vi "Main.vi"(8 "error in":errorcluster, 11 "Maestro Control in":refnum<class "Maestro Control.lvclass">) -> (0 "error out":errorcluster, 3 "Maestro Control out":refnum<class "Maestro Control.lvclass">)   [LabVIEW 2021, in "Maestro Control.lvclass"]
doc: "The Queued Message Handler of a Worker."
uses:
  Maestro Control.lvclass
  C:/Program Files (x86)/National Instruments/LabVIEW 2021/vi.lib/addons/_Workers/Library/Classes/Worker/Worker.lvclass
  Maestro Control.lvclass/Maestro Control.ctl
  <vilib>/addons/_Workers/Library/Classes/Worker/Worker.lvclass/Worker.ctl
  UI State.ctl
  85a54a2c-5f55-4a01-b73e-4297187ed6bb.vi
  85a54a2c-5f55-4a01-b73e-4297187ed6bb.vi/659df739-fa42-474c-bf03-f9ba45f35773.vi
  Maestro Acq/Maestro Acq.lvclass
  Maestro Data Logg/Maestro Data Logg.lvclass
  <userlib>/LV-TOML/lib/Parse TOML String.vi
  <userlib>/LV-TOML/lib/TOML to LabVIEW.vi
  <vilib>/addons/_Workers/Library/Classes/Message/Enqueue Message to Self v2.vi
  <userlib>/LV-TOML/lib/Write TOML File (TOML).vi
  <vilib>/addons/_Workers/Library/Classes/Message/Enqueue Message to Queue.vi
  Initialization Data.ctl
  <vilib>/addons/_Workers/Library/Classes/Worker/Worker.lvclass
  <vilib>/addons/_Workers/Debugger/Debug Client/Debug Client.lvlib
  <vilib>/addons/_Workers/Library/Classes/Message/Message.lvclass
  <userlib>/LV-TOML/lib/LV-TOML.lvlib
  C:/Program Files (x86)/National Instruments/LabVIEW 2021/vi.lib/addons/_Workers/Library/Classes/Workers Object/Workers Object.lvclass
  C:/Users/flepetit/Desktop/Gentec-maestro-Labview/Workers/Maestro Control/Maestro Control.lvclass
  C:/Users/flepetit/Desktop/Gentec-maestro-Labview/Workers/Maestro Acq/Maestro Acq.lvclass
  C:/Users/flepetit/Desktop/Gentec-maestro-Labview/Workers/Maestro Data Logg/Maestro Data Logg.lvclass
panel:
  in  "Activer les Stats":bool
  out "Maestro Online":bool
  in  "disconnect":bool
  in  "connect":bool
  in  "Port":i16
  in  "Adress(ip)":string
  out "Datas":waveform(dbl)[](graph)
  in  "délai d'acq.(ms)":i32
  in  "Log File Path":path
  out "Puiss.":dbl format="%#_6e"
  in  "Stop":bool
  in  "Start":bool
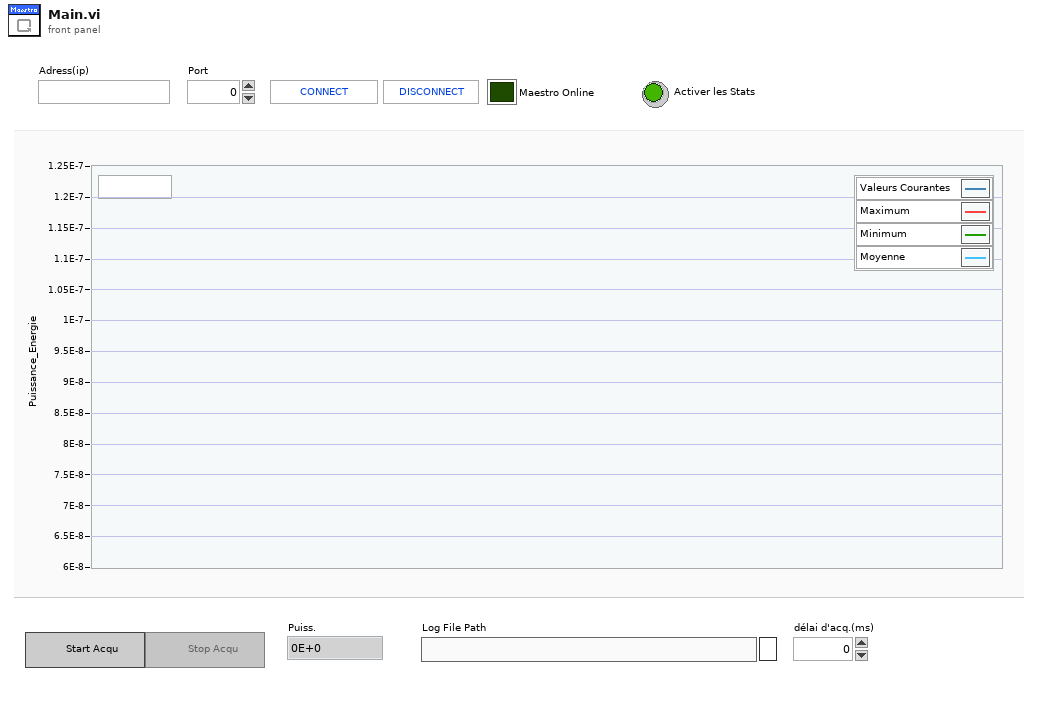
[diagram p1: front panel]
types:
  T1 = cluster{"Tps(s)":dbl[], "Puiss.":dbl, "Waveform":waveform(dbl)[]}
  T2 = enum16{"open", "replace", "create", "open or create", "replace or create", "replace or create with confirmation"}
  T3 = typedef "Maestro Control.lvclass/Initialization Data.ctl" = cluster{"String":string}
  T4 = typedef "Maestro Control.lvclass/UI State.ctl" = enum16{"Idle", "Acquiring and Logging", "Waiting for Exit", "Waiting for Exit (Acq Stopped)", "Waiting for Exit (Log Stopped)", "Waiting for Stop", "Waiting for Stop (Acq Stopped)", "Waiting for Stop (Log Stopped)"}
  T5 = typedef "Maestro Acq.lvclass/Hardware Maestro Config.ctl" = cluster{"Adress(ip)":string, "Port":i16, "Log File Base Path":path, "délai d'acq.(ms)":i32, "Activer les Stats":bool}
  T6 = typedef "Workers.lvlib/Case Label.ctl" = string
  T7 = typedef "LV-TOML.lvlib/TOML Value.ctl" = cluster{"type":enum16{"Table", "Array", "String", "Integer", "Float", "Boolean", "Offset Date-Time", "Local Date-Time", "Local Date", "Local Time", "Path"}, "value":variant}
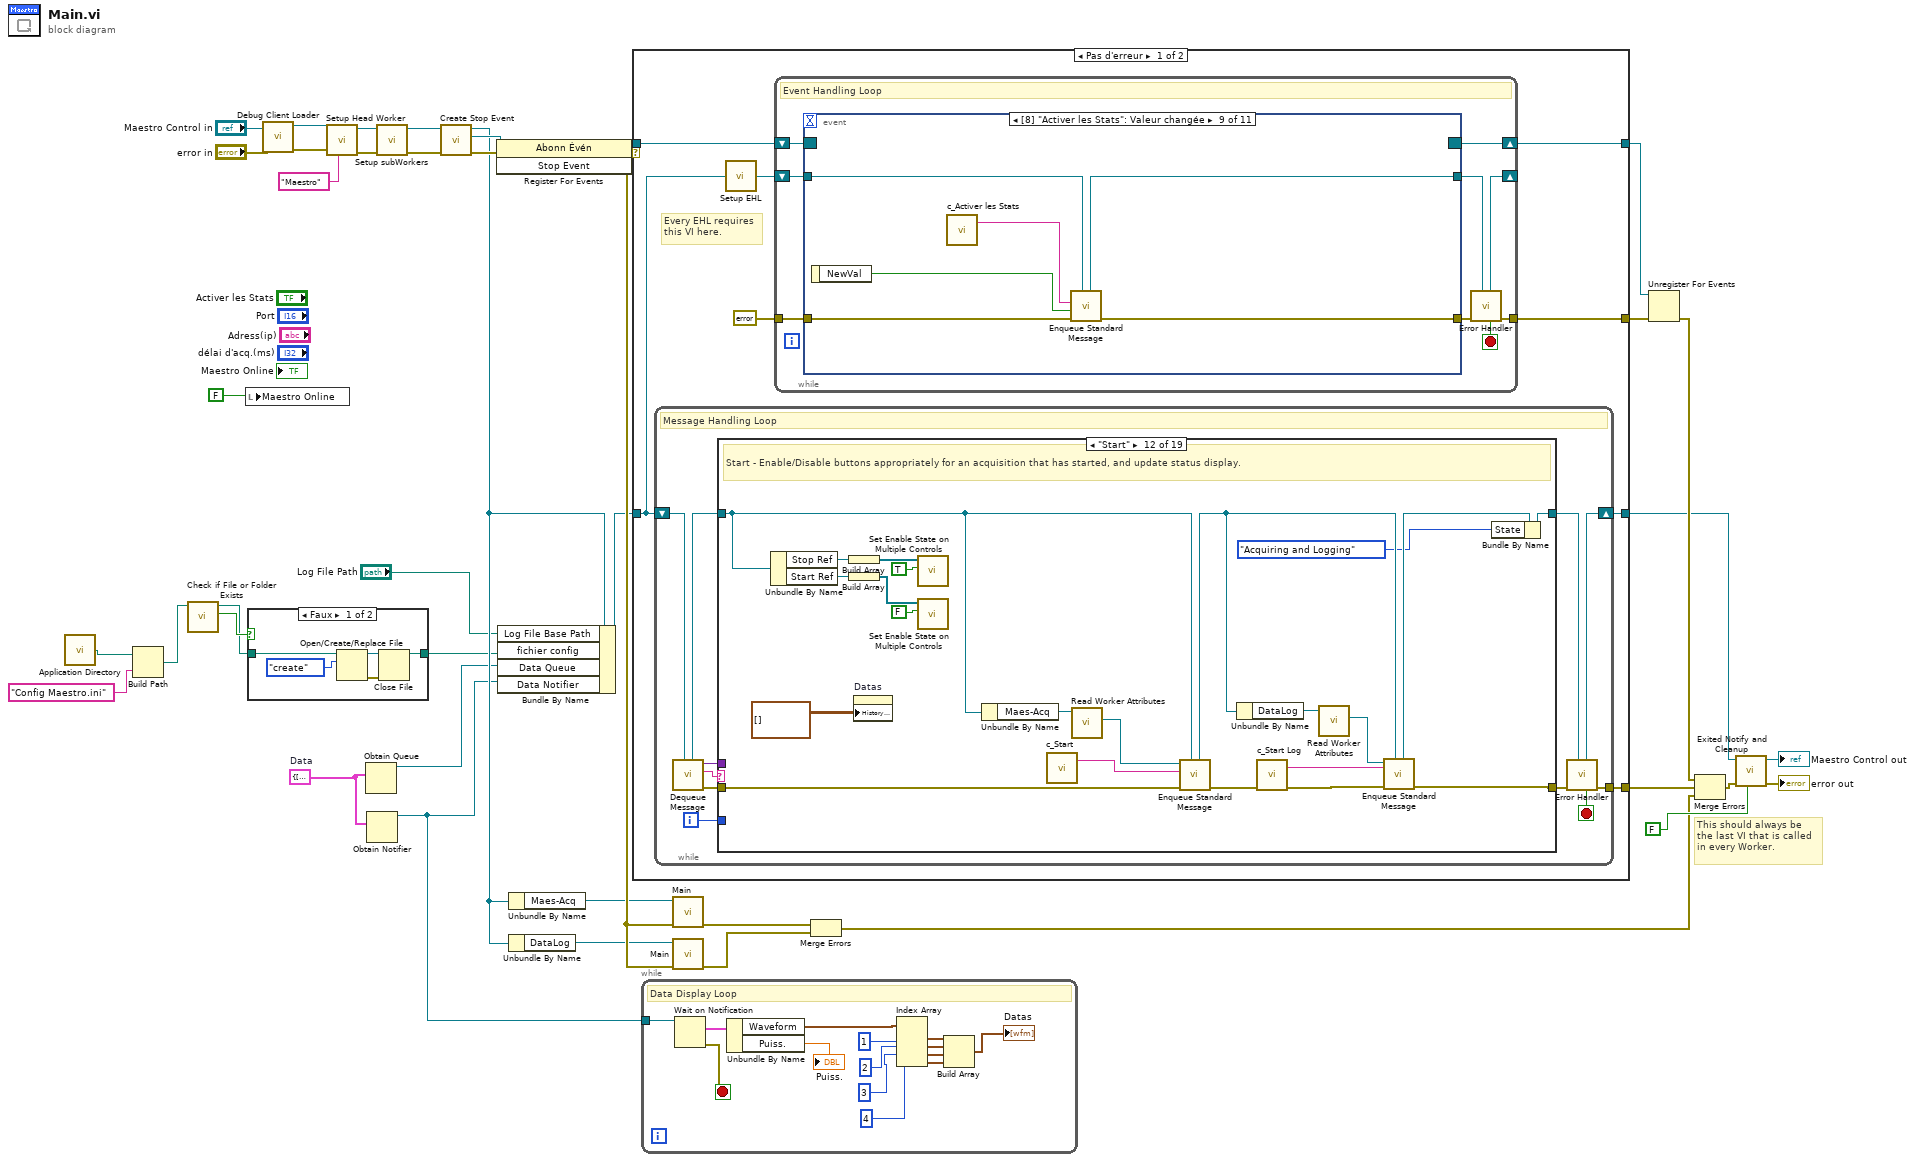
[diagram p0: block diagram]
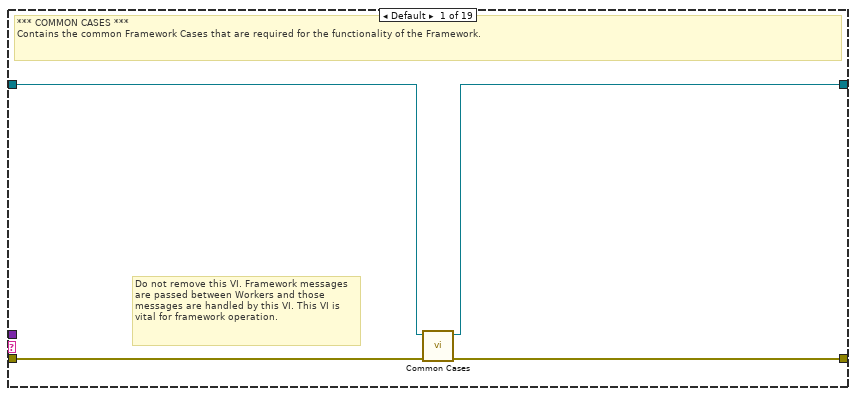
[diagram p3: hidden frame]
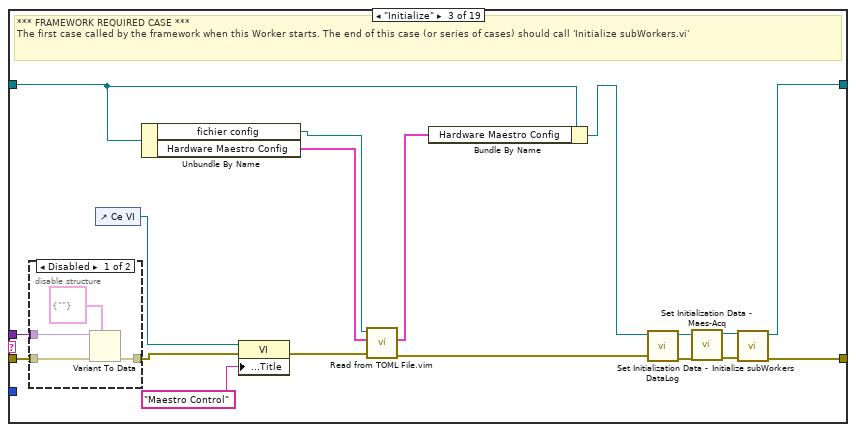
[diagram p5: hidden frame]
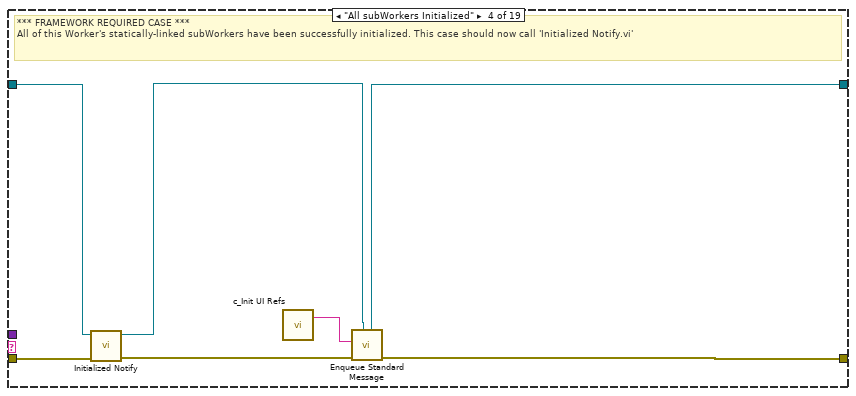
[diagram p7: hidden frame]
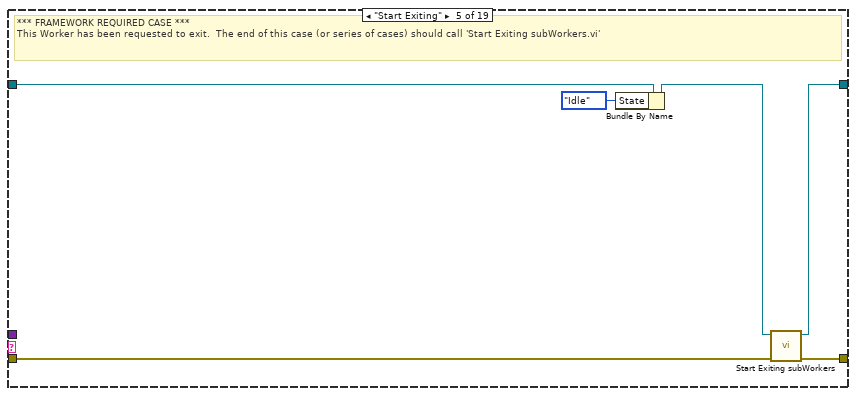
[diagram p8: hidden frame]
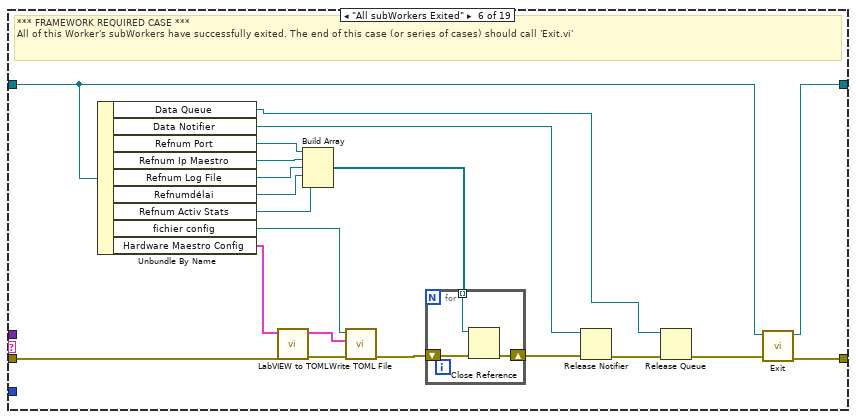
[diagram p9: hidden frame]
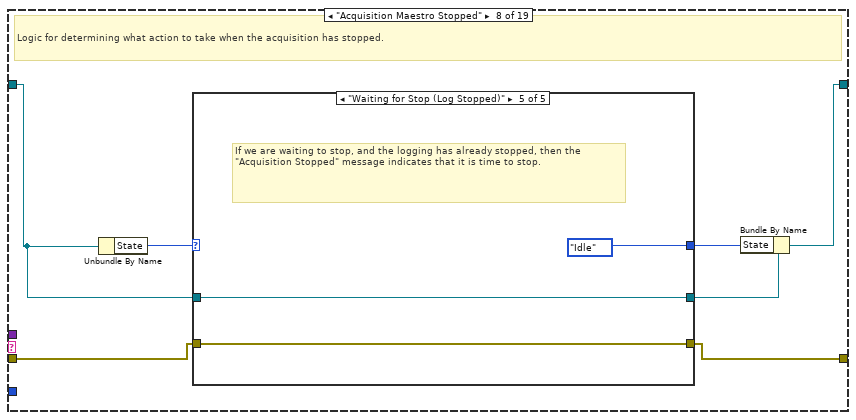
[diagram p11: hidden frame]
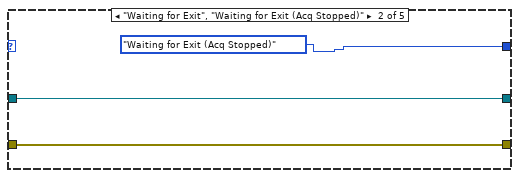
[diagram p13: hidden frame]
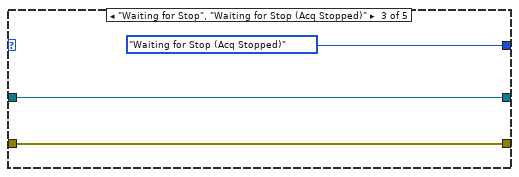
[diagram p14: hidden frame]
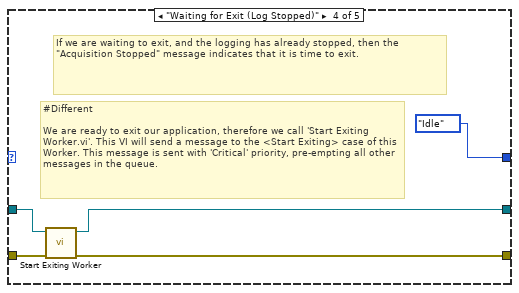
[diagram p15: hidden frame]
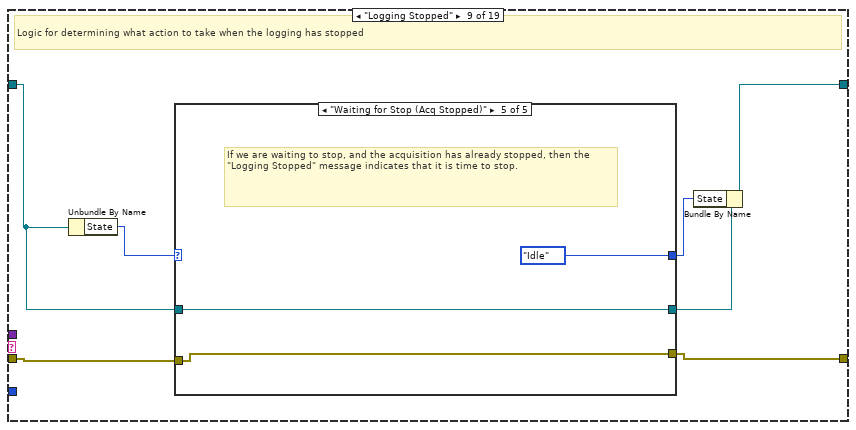
[diagram p16: hidden frame]
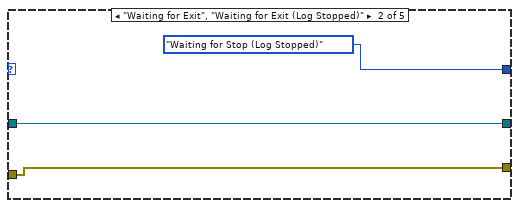
[diagram p18: hidden frame]
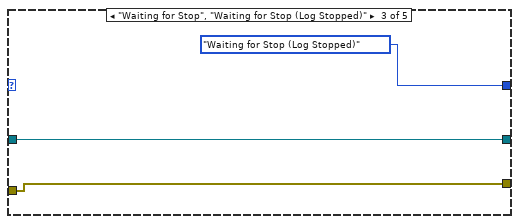
[diagram p19: hidden frame]
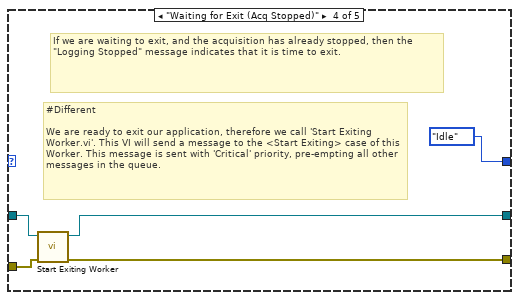
[diagram p20: hidden frame]
diagram:
  w4 = T1 {"Tps(s)"=[], "Puiss."=0.0, "Waveform"=[]}  # Data
  # "This should always be the last VI that is called in every Worker."
  n1 = call <vilib>:"Application Directory.vi"() -> ("Application Directory"=w11:path)
  n2 = Build Path(base path=w11, name or relative path="Config Maestro.ini") -> (appended path=w10:path)
  n3 = call <vilib>:"Check if File or Folder Exists.vi"("path"=w10) -> ("file or folder exists?"=w9:bool, "dup path"=w8:path)  [unwired: 8 in, 1 out]
  n4 = local write "Maestro Online"(FALSE ("connect")) -> ()
  n5 = case "Structure Condition" shown="Faux" w9 {
    tunnel: w8 -> [w45 w46]
    tunnel: [w42 w46] -> w6
    frame False {
      n6 = Open/Create/Replace File(file path (use dialog)=w45, operation (0:open)=T2."create" ("opération (0 : open)")) -> (refnum out=w44:refnum<file>, error out=w43:errorcluster)  [unwired: 4 in, 1 out]
      n7 = Close File(refnum=w44, error in=w43) -> (path=w42:path)  [unwired: 1 out]
    }
    frame True {
    }
  }
  n8 = call <vilib>:"Debug Client Loader.vi"("error in (no error)"="error in", "Worker"="Maestro Control in") -> ("error out"=w19:errorcluster, "Worker out"=w20:refnum<class "Maestro Control.lvclass">)  [unwired: 8 in]
  n9 = call-dynamic "Setup Head Worker.vi"("Worker Alias"="Maestro", "error in"=w19, "Worker"=w20) -> ("error out"=w15:errorcluster, "Worker out"=w18:refnum<class "Maestro Control.lvclass">)  [unwired: 7 in]
  n10 = Obtain Queue(element data type=w4) -> (queue out=w3:refnum<queue>)  [unwired: 4 in, 2 out]
  n11 = Obtain Notifier(notification data type=w4) -> (notifier out=w2:refnum<notifier>)  [unwired: 3 in, 2 out]
  n12 = call "Setup subWorkers.vi"("error in"=w15, "Maestro Control in"=w18) -> ("error out"=w16:errorcluster, "Maestro Control out"=w17:refnum<class "Maestro Control.lvclass">)  [unwired: 8 in]
  n13 = call-dynamic "Create Stop Event.vi"("error in"=w16, "Worker"=w17) -> ("error out"=w35:errorcluster, "Stop Event"=w32:refnum<user-event>, "Worker out"=w29:refnum<class "Maestro Control.lvclass">)  [unwired: 7 in]
  n14 = register-events(error in=w35, w32) -> (reference out=w34:refnum<event-registration>, error out=w28:errorcluster)  [unwired: 1 in]
  n15 = Bundle By Name(cluster=w29, "Log File Base Path"="Log File Path", "fichier config"=w6, "Data Queue"=w3, "Data Notifier"=w2) -> (w7:refnum<class "Maestro Control.lvclass">)
  n16 = Unbundle By Name(w29) -> ("Maes-Acq"=w23:refnum<class "Maestro Acq.lvclass">)
  n17 = Unbundle By Name(w29) -> ("DataLog"=w13:refnum<class "Maestro Data Logg.lvclass">)
  n18 = case shown="Pas d'erreur" w28 {
    tunnel: w7 -> [w49 w379]
    tunnel: [w47 w380] -> w33
    tunnel: w34 -> [w54 w381]
    tunnel: [w51 w382] -> w39
    tunnel: [w53 w381] -> w38
    tunnel: [w48 w378] -> w36
    selector: w28 -> [_ w382]
    frame No Error {
      # "Every EHL requires\nthis VI here."
      n19 = while {
        shift-right: [w63] -> w48
        shift-left: w49 -> [w65]
        tunnel: [w64] -> w47
        i -> [w55]
        stop <- w56 stop-if-true
        # "Message Handling Loop"
        n20 = call-dynamic "Dequeue Message.vi"("Worker"=w65) -> ("error out"=w62:errorcluster, "Case out"=w57:string, "Data out"=w58:variant, "Worker out"=w60:refnum<class "Maestro Control.lvclass">)  [unwired: 6 in, 1 out]
        n21 = case "Worker MHL Case Structure (DO NOT CHANGE LABEL NAME)" shown="\"Start\"" w57 {
          tunnel: w62 -> [w69 w70 w87 w100 w104 w124 w131 w138 w158 w185 w187 w207 w215 w222 w233 w245 w262 w282 w293]
          tunnel: [w68 w70 w89 w98 w107 w127 w131 w137 w157 w183 w187 w197 w210 w218 w230 w241 w249 w270 w292] -> w61
          tunnel: w60 -> [w67 w71 w81 w101 w105 w125 w132 w139 w162 w186 w188 w199 w216 w223 w234 w246 w263 w276 w302]
          tunnel: [w66 w71 w88 w96 w106 w126 w132 w135 w163 w186 w188 w191 w212 w220 w225 w240 w253 w267 w290] -> w59
          tunnel: w58 -> [_ _ w86 _ _ _ _ _ _ w184 _ _ w214 w221 w232 w244 w261 _ _]
          tunnel: w55 -> [_ _ _ _ _ _ _ _ _ _ _ _ _ _ _ _ _ _ _]
          frame Default {
            # "Do not remove this VI. Framework messages are passed between Workers and those messages are handled by this VI. This VI is vital for framework operation."
            # "*** COMMON CASES ***\nContains the common Framework Cases that are required for the functionality of the Framework."
            n22 = call-dynamic "Common Cases.vi"("error in"=w69, "Worker in"=w67) -> ("error out"=w68:errorcluster, "Worker out"=w66:refnum<class "Maestro Control.lvclass">)  [unwired: 8 in]
          }
          frame "------ FRAMEWORK REQUIRED CASES ------" {
            # "Start of Framework Required Cases"
          }
          frame "Initialize" {
            # "*** FRAMEWORK REQUIRED CASE ***\nThe first case called by the framework when this Worker starts. The end of this case (or series of cases) should call 'Initialize subWorkers.vi'"
            n23 = disable-structure shown="Disabled" {
              disable-tunnel: w87 -> [w93 w94]
              disable-tunnel: [w92 w94] -> w75
              disable-tunnel: w86 -> [w91 _]
              frame Disabled {
                n24 = Variant To Data(error in=w93, type=T3 {"String"=""} ("Initialization Data"), Variant=w91) -> (error out=w92:errorcluster)  [unwired: 1 out]
              }
              frame Enabled {
              }
            }
            n25 = control-ref of="Ce VI"() -> (w73:refnum<vi>)
            n26 = Unbundle By Name(w81) -> ("fichier config"=w82:path, "Hardware Maestro Config"=w83:T5)
            n27 = property class="VI"(reference=w73, error in=w75, "Front Panel.Title"="Maestro Control" ("Fenêtre face-avant:Titre")) -> (error out=w74:errorcluster)  [unwired: 1 out]
            n28 = call "Read from TOML File.vim"("error in (no error)"=w74, "Default Value"=w83, "file path (use dialog)"=w82) -> ("error out"=w76:errorcluster, "Value"=w80:T5)  [unwired: 6 in, 1 out]
            n29 = Bundle By Name(cluster=w81, "Hardware Maestro Config"=w80) -> (w79:refnum<class "Maestro Control.lvclass">)
            n30 = call "Set Initialization Data - DataLog.vi"("error in"=w76, "Maestro Control in"=w79) -> ("error out"=w77:errorcluster, "Maestro Control out"=w78:refnum<class "Maestro Control.lvclass">)  [unwired: 8 in]
            n31 = call "Set Initialization Data - Maes-Acq.vi"("error in"=w77, "Maestro Control in"=w78) -> ("error out"=w85:errorcluster, "Maestro Control out"=w84:refnum<class "Maestro Control.lvclass">)  [unwired: 8 in]
            n32 = call-dynamic "Initialize subWorkers.vi"("error in"=w85, "Worker"=w84) -> ("error out"=w89:errorcluster, "dup Worker out"=w88:refnum<class "Maestro Control.lvclass">)  [unwired: 8 in]
          }
          frame "All subWorkers Initialized" {
            # "*** FRAMEWORK REQUIRED CASE ***\nAll of this Worker's statically-linked subWorkers have been successfully initialized. This case should now call 'Initialized Notify.vi'"
            n33 = call-dynamic "Initialized Notify.vi"("error in"=w100, "Worker"=w101) -> ("error out"=w99:errorcluster, "dup Worker out"=w97:refnum<class "Maestro Control.lvclass">)  [unwired: 8 in]
            n34 = call "c_Init UI Refs.vi"() -> ("Case Label"=w95:T6)  [unwired: 1 in]
            n35 = call-poly <vilib>:"Enqueue Standard Message.vi"("Worker"=w97, "error in"=w99, "Case Label"=w95) -> ("error out"=w98:errorcluster, "dup Worker out"=w96:refnum<class "Maestro Control.lvclass">)  [unwired: 7 in]
          }
          frame "Start Exiting" {
            # "*** FRAMEWORK REQUIRED CASE ***\nThis Worker has been requested to exit.  The end of this case (or series of cases) should call 'Start Exiting subWorkers.vi'"
            n36 = Bundle By Name(cluster=w105, "State"=UI_State."Idle") -> (w103:refnum<class "Maestro Control.lvclass">)
            n37 = call-dynamic "Start Exiting subWorkers.vi"("error_in"=w104, "Worker"=w103) -> ("error out"=w107:errorcluster, "dup Worker out"=w106:refnum<class "Maestro Control.lvclass">)  [unwired: 8 in]
          }
          frame "All subWorkers Exited" {
            # "*** FRAMEWORK REQUIRED CASE ***\nAll of this Worker's subWorkers have successfully exited. The end of this case (or series of cases) should call 'Exit.vi'"
            n38 = Unbundle By Name(w125) -> ("Data Queue"=w112:refnum<queue>, "Data Notifier"=w113:refnum<notifier>, "Refnum Port"=w119:refnum<vi>, "Refnum Ip Maestro"=w118:refnum<vi>, "Refnum Log File"=w110:refnum<vi>, "Refnumdélai"=w109:refnum<vi>, "Refnum Activ Stats"=w108:refnum<vi>, "fichier config"=w111:path, "Hardware Maestro Config"=w122:T5)
            n39 = call <userlib>:"LabVIEW to TOML.vi"("error in (no error)"=w124, "LV Value"=w122) -> ("error out"=w123:errorcluster, "TOML Value"=w121:T7)  [unwired: 7 in, 1 out]
            n40 = Build Array(w119, w118, w110, w109, w108) -> (w117:refnum<vi>[])
            n41 = call-poly <userlib>:"Write TOML File.vi"("error in (no error)"=w123, "Value"=w121, "file path (use dialog)"=w111) -> ("error out"=w120:errorcluster)  [unwired: 8 in]
            n42 = for {
              shift-right: [w129] -> w115
              shift-left: w120 -> [w130]
              tunnel: w117 -> [w128] mode=indexing
              n43 = Close Reference(reference=w128, error in (no error)=w130) -> (error out=w129:errorcluster)
            }
            n44 = Release Notifier(notifier=w113, error in (no error)=w115) -> (error out=w116:errorcluster)  [unwired: 1 in, 2 out]
            n45 = Release Queue(queue=w112, error in (no error)=w116) -> (error out=w114:errorcluster)  [unwired: 1 in, 2 out]
            n46 = call-dynamic "Exit.vi"("error_in"=w114, "Worker"=w125) -> ("error out"=w127:errorcluster, "dup Worker out"=w126:refnum<class "Maestro Control.lvclass">)  [unwired: 8 in]
          }
          frame "---------From Maestro Acq---------------------" {
            # "End of Framework Required Cases"
          }
          frame "Acquisition Maestro Stopped" {
            # "Logic for determining what action to take when the acquisition has stopped."
            n47 = Unbundle By Name(w139) -> ("State"=w133:T4)
            n48 = case shown="\"Waiting for Stop (Log Stopped)\"" w133 {
              selector: w133 -> [w142 _ _ _ _]
              tunnel: [w142 UI_State."Waiting for Exit (Acq Stopped)" ("UI State") UI_State."Waiting for Stop (Acq Stopped)" ("UI State") UI_State."Idle" ("UI State") UI_State."Idle" ("UI State")] -> w134
              tunnel: [w141 w145 w148 w151 w156] -> w137
              tunnel: w138 -> [w141 w145 w148 w152 w156]
              tunnel: w139 -> [w140 w144 w147 w153 w155]
              tunnel: [w140 w144 w147 w150 w155] -> w136
              frame Default {
              }
              frame "Waiting for Exit", "Waiting for Exit (Acq Stopped)" {
              }
              frame "Waiting for Stop", "Waiting for Stop (Acq Stopped)" {
              }
              frame "Waiting for Exit (Log Stopped)" {
                # "#Different\n\nWe are ready to exit our application, therefore we call 'Start Exiting Worker.vi'. This VI will send a message to the <Start Exiting> case of this Worker. This message is sent with 'Critical' priority, pre-empting all other messages in the queue."
                # "If we are waiting to exit, and the logging has already stopped, then the \"Acquisition Stopped\" message indicates that it is time to exit."
                n49 = call-dynamic "Start Exiting Worker.vi"("error in"=w152, "Worker"=w153) -> ("error out"=w151:errorcluster, "dup Worker out"=w150:refnum<class "Maestro Control.lvclass">)  [unwired: 8 in]
              }
              frame "Waiting for Stop (Log Stopped)" {
                # "If we are waiting to stop, and the logging has already stopped, then the \"Acquisition Stopped\" message indicates that it is time to stop."
              }
            }
            n50 = Bundle By Name(cluster=w136, "State"=w134) -> (w135:refnum<class "Maestro Control.lvclass">)
          }
          frame "Logging Stopped" {
            # "Logic for determining what action to take when the logging has stopped"
            n51 = Unbundle By Name(w162) -> ("State"=w159:T4)
            n52 = case shown="\"Waiting for Stop (Acq Stopped)\"" w159 {
              selector: w159 -> [w166 _ _ _ _]
              tunnel: [w166 UI_State."Waiting for Stop (Log Stopped)" ("UI State") UI_State."Waiting for Stop (Log Stopped)" ("UI State") UI_State."Idle" ("UI State") UI_State."Idle" ("UI State")] -> w160
              tunnel: [w164 w168 w171 w176 w178] -> w157
              tunnel: w162 -> [w165 w169 w172 w177 w180]
              tunnel: [w165 w169 w172 w175 w180] -> w161
              tunnel: w158 -> [w164 w168 w171 w173 w178]
              frame Default {
              }
              frame "Waiting for Exit", "Waiting for Exit (Log Stopped)" {
              }
              frame "Waiting for Stop", "Waiting for Stop (Log Stopped)" {
              }
              frame "Waiting for Exit (Acq Stopped)" {
                # "#Different\n\nWe are ready to exit our application, therefore we call 'Start Exiting Worker.vi'. This VI will send a message to the <Start Exiting> case of this Worker. This message is sent with 'Critical' priority, pre-empting all other messages in the queue."
                # "If we are waiting to exit, and the acquisition has already stopped, then the \"Logging Stopped\" message indicates that it is time to exit."
                n53 = call-dynamic "Start Exiting Worker.vi"("error in"=w173, "Worker"=w177) -> ("error out"=w176:errorcluster, "dup Worker out"=w175:refnum<class "Maestro Control.lvclass">)  [unwired: 8 in]
              }
              frame "Waiting for Stop (Acq Stopped)" {
                # "If we are waiting to stop, and the acquisition has already stopped, then the \"Logging Stopped\" message indicates that it is time to stop."
              }
            }
            n54 = Bundle By Name(cluster=w161, "State"=w160) -> (w163:refnum<class "Maestro Control.lvclass">)
          }
          frame "Maestro Online" {
            # "Status de la connection du maestro"
            n55 = Variant To Data(error in=w185, type=TRUE, Variant=w184) -> (data=w181:bool, error out=w183:errorcluster)
            n56 = local write "Maestro Online"(w181) -> ()
          }
          frame "----------------------Himself----------------------" {
            # "End of Framework Required Cases"
          }
          frame "Start" {
            # "Start - Enable/Disable buttons appropriately for an acquisition that has started, and update status display."
            n57 = Unbundle By Name(w199) -> ("Stop Ref"=w201:refnum<vi>, "Start Ref"=w200:refnum<vi>)
            n58 = Build Array(w201) -> (w202:refnum<vi>[])
            n59 = Build Array(w200) -> (w205:refnum<vi>[])
            n60 = property on="Datas" class="GraphDér (strict)"("History Data"=waveform(dbl)[][] [] ("Données d'historique")) -> ()  [unwired: 2 in, 2 out]
            n61 = call "Set Enable State on Multiple Controls.vi"("Enable?"=TRUE, "Controls"=w202) -> ()  [unwired: 10 in]
            n62 = call "Set Enable State on Multiple Controls.vi"("Enable?"=FALSE, "Controls"=w205) -> ()  [unwired: 10 in]
            n63 = Unbundle By Name(w199) -> ("Maes-Acq"=w209:refnum<class "Maestro Acq.lvclass">)
            n64 = call "c_Start.vi"() -> ("Case Label"=w206:T6)  [unwired: 1 in]
            n65 = call-poly <vilib>:"Read Worker Attributes.vi"("Worker"=w209) -> ("Message Queue out"=w208:refnum<class "Message Queue.lvclass">)  [unwired: 9 in, 1 out]
            n66 = call-poly <vilib>:"Enqueue Standard Message.vi"("Worker"=w199, "error in"=w207, "Case Label"=w206, "Message Queue"=w208) -> ("error out"=w198:errorcluster, "dup Worker out"=w194:refnum<class "Maestro Control.lvclass">)  [unwired: 5 in, 1 out]
            n67 = Unbundle By Name(w194) -> ("DataLog"=w193:refnum<class "Maestro Data Logg.lvclass">)
            n68 = call "c_Start Log.vi"() -> ("Case Label"=w195:T6)  [unwired: 1 in]
            n69 = call-poly <vilib>:"Read Worker Attributes.vi"("Worker"=w193) -> ("Message Queue out"=w192:refnum<class "Message Queue.lvclass">)  [unwired: 9 in, 1 out]
            n70 = call-poly <vilib>:"Enqueue Standard Message.vi"("Worker"=w194, "error in"=w198, "Case Label"=w195, "Message Queue"=w192) -> ("error out"=w197:errorcluster, "dup Worker out"=w196:refnum<class "Maestro Control.lvclass">)  [unwired: 5 in, 1 out]
            n71 = Bundle By Name(cluster=w196, "State"=UI_State."Acquiring and Logging") -> (w191:refnum<class "Maestro Control.lvclass">)
          }
          frame "Update adress ip" {
            # "Update adresse ip du maestro"
            n72 = Variant To Data(error in=w215, type="", Variant=w214) -> (data=w211:string, error out=w210:errorcluster)
            n73 = Bundle By Name(cluster=w216, "Adress(ip)"=w211) -> (w212:refnum<class "Maestro Control.lvclass">)
          }
          frame "Update Port" {
            # "Update port TCP"
            n74 = Variant To Data(error in=w222, type=i16 0, Variant=w221) -> (data=w219:i16, error out=w218:errorcluster)
            n75 = Bundle By Name(cluster=w223, "Port"=w219) -> (w220:refnum<class "Maestro Control.lvclass">)
          }
          frame "Update Log File" {
            # "#Updating_log_file_path"
            n76 = Variant To Data(error in=w233, type=path "" ("Settings Maestro.Logging Configuration.Log File Base Path"), Variant=w232) -> (data=w224:path, error out=w230:errorcluster)
            n77 = Bundle By Name(cluster=w234, "Log File Base Path"=w224) -> (w226:refnum<class "Maestro Control.lvclass">)
            n78 = Unbundle By Name(w226) -> ("DataLog"=w228:refnum<class "Maestro Data Logg.lvclass">)
            n79 = call "c_Log file path Update.vi"() -> ("Case Label"=w229:T6)  [unwired: 1 in]
            n80 = call <vilib>:"Read Queue.vi"("Worker"=w228) -> ("Message Queue out"=w227:refnum<class "Message Queue.lvclass">)  [unwired: 9 in, 1 out]
            n81 = call-poly <vilib>:"Enqueue Standard Message.vi"("Worker"=w226, "Data"=w224, "Case Label"=w229, "Message Queue"=w227) -> ("dup Worker out"=w225:refnum<class "Maestro Control.lvclass">)  [unwired: 5 in, 2 out]
          }
          frame "Update délai" {
            # "Update du délai en ms"
            n82 = Variant To Data(error in=w245, type=0 ("délai d'acq.(ms) 2"), Variant=w244) -> (data=w235:i32, error out=w242:errorcluster)
            n83 = Bundle By Name(cluster=w246, "délai d'acq.(ms)"=w235) -> (w239:refnum<class "Maestro Control.lvclass">)
            n84 = Unbundle By Name(w239) -> ("Maes-Acq"=w238:refnum<class "Maestro Acq.lvclass">)
            n85 = call "c_Change délai.vi"() -> ("Case Label"=w236:T6)  [unwired: 1 in]
            n86 = call <vilib>:"Read Queue.vi"("Worker"=w238) -> ("Message Queue out"=w237:refnum<class "Message Queue.lvclass">)  [unwired: 9 in, 1 out]
            n87 = call-poly <vilib>:"Enqueue Standard Message.vi"("Worker"=w239, "error in"=w242, "Data"=w235, "Case Label"=w236, "Message Queue"=w237) -> ("error out"=w241:errorcluster, "dup Worker out"=w240:refnum<class "Maestro Control.lvclass">)  [unwired: 4 in, 1 out]
          }
          frame "Activer les Stats" {
            # "Active les statistiques du gentec maestro"
            n88 = Variant To Data(error in=w262, type=FALSE, Variant=w261) -> (data=w248:bool, error out=w256:errorcluster)
            n89 = Bundle By Name(cluster=w263, "Activer les Stats"=w248) -> (w257:refnum<class "Maestro Control.lvclass">)
            n90 = Unbundle By Name(w257) -> ("Maes-Acq"=w259:refnum<class "Maestro Acq.lvclass">)
            n91 = call "c_Activer stats.vi"() -> ("Case Label"=w255:T6)  [unwired: 1 in]
            n92 = call <vilib>:"Read Queue.vi"("Worker"=w259) -> ("Message Queue out"=w258:refnum<class "Message Queue.lvclass">)  [unwired: 9 in, 1 out]
            n93 = call-poly <vilib>:"Enqueue Standard Message.vi"("Worker"=w257, "error in"=w256, "Data"=w248, "Case Label"=w255, "Message Queue"=w258) -> ("error out"=w250:errorcluster, "dup Worker out"=w252:refnum<class "Maestro Control.lvclass">)  [unwired: 4 in, 1 out]
            n94 = Unbundle By Name(w252) -> ("DataLog"=w254:refnum<class "Maestro Data Logg.lvclass">)
            n95 = call "c_Activer stats.vi"() -> ("Case Label"=w247:T6)  [unwired: 1 in]
            n96 = call <vilib>:"Read Queue.vi"("Worker"=w254) -> ("Message Queue out"=w251:refnum<class "Message Queue.lvclass">)  [unwired: 9 in, 1 out]
            n97 = call-poly <vilib>:"Enqueue Standard Message.vi"("Worker"=w252, "error in"=w250, "Data"=w248, "Case Label"=w247, "Message Queue"=w251) -> ("error out"=w249:errorcluster, "dup Worker out"=w253:refnum<class "Maestro Control.lvclass">)  [unwired: 4 in, 1 out]
          }
          frame "Stop" {
            # "Stop - Enable/Disable buttons appropriately for an acquisition that has stopped, and update status display."
            n98 = Unbundle By Name(w276) -> ("Stop Ref"=w275:refnum<vi>, "Start Ref"=w274:refnum<vi>)
            n99 = Build Array(w275) -> (w277:refnum<vi>[])
            n100 = Build Array(w274) -> (w280:refnum<vi>[])
            n101 = call "Set Enable State on Multiple Controls.vi"("Enable?"=TRUE, "Controls"=w280) -> ()  [unwired: 10 in]
            n102 = call "Set Enable State on Multiple Controls.vi"("Enable?"=FALSE, "Controls"=w277) -> ()  [unwired: 10 in]
            n103 = Unbundle By Name(w276) -> ("Maes-Acq"=w284:refnum<class "Maestro Acq.lvclass">)
            n104 = call "c_Stop.vi"() -> ("Case Label"=w281:T6)  [unwired: 1 in]
            n105 = call-poly <vilib>:"Read Worker Attributes.vi"("Worker"=w284) -> ("Message Queue out"=w283:refnum<class "Message Queue.lvclass">)  [unwired: 9 in, 1 out]
            n106 = call-poly <vilib>:"Enqueue Standard Message.vi"("Worker"=w276, "error in"=w282, "Case Label"=w281, "Message Queue"=w283) -> ("error out"=w271:errorcluster, "dup Worker out"=w266:refnum<class "Maestro Control.lvclass">)  [unwired: 5 in, 1 out]
            n107 = Unbundle By Name(w266) -> ("State"=w265:T4)
            n108 = Unbundle By Name(w266) -> ("DataLog"=w273:refnum<class "Maestro Data Logg.lvclass">)
            n109 = call "c_Stop Log.vi"() -> ("Case Label"=w268:T6)  [unwired: 1 in]
            n110 = case shown="\"Waiting for Exit\"" w265 {
              selector: w265 -> [_ w286]
              tunnel: [UI_State."Waiting for Stop" ("State") w286] -> w264
              frame Default {
              }
              frame "Waiting for Exit" {
              }
            }
            n111 = call-poly <vilib>:"Read Worker Attributes.vi"("Worker"=w273) -> ("Message Queue out"=w272:refnum<class "Message Queue.lvclass">)  [unwired: 9 in, 1 out]
            n112 = call-poly <vilib>:"Enqueue Standard Message.vi"("Worker"=w266, "error in"=w271, "Case Label"=w268, "Message Queue"=w272) -> ("error out"=w270:errorcluster, "dup Worker out"=w269:refnum<class "Maestro Control.lvclass">)  [unwired: 5 in, 1 out]
            n113 = Bundle By Name(cluster=w269, "State"=w264) -> (w267:refnum<class "Maestro Control.lvclass">)
          }
          frame "Init UI Refs" {
            # "Init UI Refs - Store control references for UI controls.  Also enable/disable controls appropriately."
            n114 = control-ref of="délai d'acq.(ms)"() -> (w288:refnum<vi>)
            n115 = control-ref of="Log File Path"() -> (w289:refnum<vi>)
            n116 = control-ref of="Activer les Stats"() -> (w287:refnum<vi>)
            n117 = control-ref of="Port"() -> (w294:refnum<vi>)
            n118 = control-ref of="Start"() -> (w301:refnum<vi>)
            n119 = control-ref of="Adress(ip)"() -> (w295:refnum<vi>)
            n120 = control-ref of="Stop"() -> (w298:refnum<vi>)
            n121 = Bundle By Name(cluster=w302, "Start Ref"=w301, "Stop Ref"=w298, "Refnum Ip Maestro"=w295, "Refnum Port"=w294, "Refnum Log File"=w289, "Refnumdélai"=w288, "Refnum Activ Stats"=w287) -> (w291:refnum<class "Maestro Control.lvclass">)
            n122 = Build Array(w298) -> (w296:refnum<vi>[])
            n123 = Build Array(w301) -> (w300:refnum<vi>[])
            n124 = call "Set Enable State on Multiple Controls.vi"("Enable?"=TRUE, "Controls"=w300) -> ()  [unwired: 10 in]
            n125 = call "Set Enable State on Multiple Controls.vi"("Enable?"=FALSE, "Controls"=w296) -> ()  [unwired: 10 in]
            n126 = call "Show value.vi"("error in (no error)"=w293, "Maestro Control en entrée"=w291) -> ("error out"=w292:errorcluster, "Maestro Control en sortie"=w290:refnum<class "Maestro Control.lvclass">)  [unwired: 8 in]
          }
        }
        n127 = call-dynamic "Error Handler.vi"("Worker"=w59, "error_in"=w61) -> ("error out"=w64:errorcluster, "Stop Loop"=w56:bool, "Worker out"=w63:refnum<class "Maestro Control.lvclass">)  [unwired: 7 in]
      }
      n128 = call-dynamic "Setup EHL.vi"("Worker"=w49) -> ("Worker out"=w50:refnum<class "Maestro Control.lvclass">)  [unwired: 14 in]
      n129 = while "Event Handling Loop" {
        shift-right: [w311] -> w53
        shift-left: w54 -> [w310]
        tunnel: [w306] -> w51
        tunnel: errorcluster {"status"=FALSE, "code"=0, "source"=""} ("error constant") -> [w308]
        shift-right: [w304] -> _
        shift-left: w50 -> [w309]
        stop <- w303 stop-if-true
        # "Event Handling Loop"
        n130 = event shown="[8] \"Activer les Stats\": Valeur changée" {
          selector: w310 -> [_ _ _ _ _ _ _ _ _ _ _]
          dyn-events: [_ _ _ _ _ _ _ _ _ _ _] -> w311
          timeout: _ -> [_ _ _ _ _ _ _ _ _ _ _]
          tunnel: [w315 w322 w327 w332 w338 w344 w350 w354 w360 w369 w376] -> w307
          tunnel: w308 -> [w316 w321 w328 w333 w339 w345 w351 w355 w361 w370 w377]
          tunnel: w309 -> [w314 w320 w326 w331 w337 w343 w349 w357 w363 w366 w373]
          tunnel: [w313 w319 w325 w330 w336 w342 w348 w356 w362 w365 w372] -> w305
          event User Event {
            # "This case and its contents must always be included in every EHL that you use, so that the framework can automatically stop the EHL."
            # "EHL Stop Event. This EHL exits from this case."
            n131 = event-data() -> ("Stop Event Data"=w312:variant)  [unwired: 1 in]
            n132 = call <vilib>:"EHL Stop - EHL Case.vi"("error in"=w316, "Stop Event Data"=w312, "Worker"=w314) -> ("error out"=w315:errorcluster, "Worker out"=w313:refnum<class "Maestro Control.lvclass">)  [unwired: 7 in]
          }
          event Panel Close? {
            # "Use this VI when you want to exit this Worker. This VI will call the Start Exiting case of this Worker. This is the correct way to exit your Worker."
            # "Calls the Start Exiting case of this Worker. This will start the exiting sequence of this Worker."
            n133 = event-data() -> ()  [unwired: 1 in, 1 out]
            n134 = call <vilib>:"Read Queue.vi"("Worker"=w320) -> ("Message Queue out"=w317:refnum<class "Message Queue.lvclass">, "dup Worker out"=w318:refnum<class "Maestro Control.lvclass">)  [unwired: 9 in]
            n135 = call-dynamic "Worker Start Exiting.vi"("error_in"=w321, "Message Queue"=w317, "Worker"=w318) -> ("error out"=w322:errorcluster, "dup Worker out"=w319:refnum<class "Maestro Control.lvclass">)  [unwired: 7 in]
            n136 = event-data ("Nœud de filtre d'événements")("Discard?"=TRUE) -> ()  [unwired: 1 in, 1 out]
          }
          event "Start": Value Change {
            n137 = event-data() -> ()  [unwired: 1 in, 1 out]
            n138 = call "c_Start.vi"() -> ("Case Label"=w324:T6)  [unwired: 1 in]
            n139 = call-poly <vilib>:"Enqueue Standard Message.vi"("Worker"=w326, "error in"=w328, "Case Label"=w324) -> ("error out"=w327:errorcluster, "dup Worker out"=w325:refnum<class "Maestro Control.lvclass">)  [unwired: 7 in]
          }
          event "Stop": Value Change {
            n140 = event-data() -> ()  [unwired: 1 in, 1 out]
            n141 = call "c_Stop.vi"() -> ("Case Label"=w329:T6)  [unwired: 1 in]
            n142 = call-poly <vilib>:"Enqueue Standard Message.vi"("Worker"=w331, "error in"=w333, "Case Label"=w329) -> ("error out"=w332:errorcluster, "dup Worker out"=w330:refnum<class "Maestro Control.lvclass">)  [unwired: 7 in]
          }
          event "Log File Path": Value Change {
            n143 = event-data() -> ("NewVal"=w334:path)  [unwired: 1 in]
            n144 = call "c_Update Log File.vi"() -> ("Case Label"=w335:T6)  [unwired: 1 in]
            n145 = call-poly <vilib>:"Enqueue Standard Message.vi"("Worker"=w337, "error in"=w339, "Data"=w334, "Case Label"=w335) -> ("error out"=w338:errorcluster, "dup Worker out"=w336:refnum<class "Maestro Control.lvclass">)  [unwired: 6 in]
          }
          event "Adress(ip)": Value Change {
            n146 = event-data() -> ("NewVal"=w340:string)  [unwired: 1 in]
            n147 = call "c_Update adress ip.vi"() -> ("Case Label"=w341:T6)  [unwired: 1 in]
            n148 = call-poly <vilib>:"Enqueue Standard Message.vi"("Worker"=w343, "error in"=w345, "Data"=w340, "Case Label"=w341) -> ("error out"=w344:errorcluster, "dup Worker out"=w342:refnum<class "Maestro Control.lvclass">)  [unwired: 6 in]
          }
          event "Port": Value Change {
            n149 = event-data() -> ("NewVal"=w346:i16)  [unwired: 1 in]
            n150 = call "c_Update Port.vi"() -> ("Case Label"=w347:T6)  [unwired: 1 in]
            n151 = call-poly <vilib>:"Enqueue Standard Message.vi"("Worker"=w349, "error in"=w351, "Data"=w346, "Case Label"=w347) -> ("error out"=w350:errorcluster, "dup Worker out"=w348:refnum<class "Maestro Control.lvclass">)  [unwired: 6 in]
          }
          event "délai d'acq.(ms)": Value Change {
            n152 = event-data() -> ("NewVal"=w352:i32)  [unwired: 1 in]
            n153 = call "c_Update délai.vi"() -> ("Case Label"=w353:T6)  [unwired: 1 in]
            n154 = call-poly <vilib>:"Enqueue Standard Message.vi"("Worker"=w357, "error in"=w355, "Data"=w352, "Case Label"=w353) -> ("error out"=w354:errorcluster, "dup Worker out"=w356:refnum<class "Maestro Control.lvclass">)  [unwired: 6 in]
          }
          event "Activer les Stats": Value Change {
            n155 = event-data() -> ("NewVal"=w359:bool)  [unwired: 1 in]
            n156 = call "c_Activer les Stats.vi"() -> ("Case Label"=w358:T6)  [unwired: 1 in]
            n157 = call-poly <vilib>:"Enqueue Standard Message.vi"("Worker"=w363, "error in"=w361, "Data"=w359, "Case Label"=w358) -> ("error out"=w360:errorcluster, "dup Worker out"=w362:refnum<class "Maestro Control.lvclass">)  [unwired: 6 in]
          }
          event "connect": Value Change {
            n158 = event-data() -> ()  [unwired: 1 in, 1 out]
            n159 = Unbundle By Name ("Désassembler par nom")(w366) -> ("Maes-Acq"=w367:refnum<class "Maestro Acq.lvclass">)
            n160 = call "c_Connect Maestro.vi"() -> ("Case Label"=w364:T6)  [unwired: 1 in]
            n161 = call <vilib>:"Read Queue.vi"("Worker"=w367) -> ("Message Queue out"=w368:refnum<class "Message Queue.lvclass">)  [unwired: 9 in, 1 out]
            n162 = call-poly <vilib>:"Enqueue Standard Message.vi"("Worker"=w366, "error in"=w370, "Case Label"=w364, "Message Queue"=w368) -> ("error out"=w369:errorcluster, "dup Worker out"=w365:refnum<class "Maestro Control.lvclass">)  [unwired: 5 in, 1 out]
          }
          event "disconnect": Value Change {
            n163 = event-data() -> ()  [unwired: 1 in, 1 out]
            n164 = Unbundle By Name ("Désassembler par nom")(w373) -> ("Maes-Acq"=w374:refnum<class "Maestro Acq.lvclass">)
            n165 = call "c_disconnect maestro.vi"() -> ("Case Label"=w371:T6)  [unwired: 1 in]
            n166 = call <vilib>:"Read Queue.vi"("Worker"=w374) -> ("Message Queue out"=w375:refnum<class "Message Queue.lvclass">)  [unwired: 9 in, 1 out]
            n167 = call-poly <vilib>:"Enqueue Standard Message.vi"("Worker"=w373, "error in"=w377, "Case Label"=w371, "Message Queue"=w375) -> ("error out"=w376:errorcluster, "dup Worker out"=w372:refnum<class "Maestro Control.lvclass">)  [unwired: 5 in, 1 out]
          }
        }
        n168 = call-dynamic "Error Handler.vi"("Worker"=w305, "error_in"=w307) -> ("error out"=w306:errorcluster, "Stop Loop"=w303:bool, "Worker out"=w304:refnum<class "Maestro Control.lvclass">)  [unwired: 7 in]
      }
    }
    frame Error {
      n169 = call-dynamic "Error Handler.vi"("Worker"=w379, "error_in"=w382) -> ("error out"=w380:errorcluster, "Worker out"=w378:refnum<class "Maestro Control.lvclass">)  [unwired: 7 in, 1 out]
    }
  }
  n170 = while "Data Display Loop" {
    tunnel: w2 -> [w396]
    stop <- w395 stop-if-true
    # "Data Display Loop"
    n171 = Wait on Notification(notifier=w396) -> (notification=w394:T1, error out=w395:errorcluster)  [unwired: 3 in, 2 out]
    n172 = Unbundle By Name(w394) -> ("Waveform"=w392:waveform(dbl)[], "Puiss."=→"Puiss.":dbl)
    n173 = Index Array(array=w392, index #1=1 ("indice"), index #2=2 ("indice"), index #3=3 ("indice"), index #4=4 ("indice")) -> (element #1=w387:waveform(dbl), element #2=w386:waveform(dbl), element #3=w385:waveform(dbl), element #4=w384:waveform(dbl))
    n174 = Build Array(w387, w386, w385, w384) -> (→"Datas":waveform(dbl)[])
  }
  n175 = call-dynamic "Main.vi"("error in"=w28, "Maestro Acq in"=w23) -> ("error out"=w25:errorcluster)  [unwired: 8 in, 1 out]
  n176 = call-dynamic "Main.vi"("error in"=w28, "Maestro Data Logg in"=w13) -> ("error out"=w14:errorcluster)  [unwired: 8 in, 1 out]
  n177 = Merge Errors(w25, w14) -> (w24:errorcluster)
  n178 = Unregister For Events(event registration refnum=w38, error in=w39) -> (error out=w40:errorcluster)
  n179 = Merge Errors ("Fusionner les erreurs")(w40, w33, w24) -> (w37:errorcluster)
  n180 = call-dynamic "Exited Notify and Cleanup.vi"("Close FP on Exit? (T)"=FALSE, "error_in"=w37, "Worker"=w36) -> ("error out"=→"error out":errorcluster, "dup Worker out"=→"Maestro Control out":refnum<class "Maestro Control.lvclass">)  [unwired: 7 in]
